vi "Autonomous Independent.vi"   [LabVIEW 2015]
doc: "This VI is called when autonomous begins, and will automatically be terminated when autonomous ends. You can carry out timed or sensor driven robot movement independently without needing to return to the caller."
uses:
  <vilib>/Rock Robotics/WPI/Relay/WPI_RelayValue.ctl
  <vilib>/Rock Robotics/WPI/Utilities/WPI_GetSetVariantRefNum.vi
  <vilib>/Rock Robotics/Network Tables/NT Read String.vi
  <vilib>/Rock Robotics/Network Tables/NT Read Number.vi
  <vilib>/Rock Robotics/Network Tables/NT Write Numeric Array.vi
panel:
  # "Be sure to right-click and choose Data Operations>>Make Current Value default if you want to save the array values with the VI"
types:
  T1 = typedef "WPI_JoystickDevRef.ctl" = cluster{"Device":T2}
  T2 = typedef "WPI_JoystickDeviceEnum.ctl" = enum16{"USB 0", "USB 1", "USB 2", "USB 3", "USB 4", "USB 5"}
  T3 = typedef "WPI_ServoDeviceRef.ctl" = cluster{"DeviceStatus":errorcluster, "PWM Channel":T4, "DeadBand":T5}
  T4 = typedef "FPGA_DIOPWMChannel.ctl" = enum8{"PWM 0", "PWM 1", "PWM 2", "PWM 3", "PWM 4", "PWM 5", "PWM 6", "PWM 7", "PWM 8", "PWM 9", "PWM MXP 0", "PWM MXP 1", "PWM MXP 2", "PWM MXP 3", "PWM MXP 4", "PWM MXP 5", "PWM MXP 6", "PWM MXP 7", "PWM MXP 8", "PWM MXP 9", "Invalid"}
  T5 = typedef "WPI_PWMDeadband.ctl" = cluster{"Name":string, "maxPositivePwm":i32, "minPositivePwm":i32, "centerPwm":i32, "maxNegativePwm":i32, "minNegativePwm":i32, "angularRange":u16}
  T6 = typedef "WPI_RelayValue.ctl" = enum16{"Off", "On", "Forward", "Reverse"}
  T7 = typedef "WPI_SwitchDevRef.ctl" = cluster{"DevStatus":errorcluster, "DIO Channel":T8, "CntIndex":T9, "Normally Closed":bool}
  T8 = typedef "FPGA_DIOChannel.ctl" = enum8{"DIO 0", "DIO 1", "DIO 2", "DIO 3", "DIO 4", "DIO 5", "DIO 6", "DIO 7", "DIO 8", "DIO 9", "DIO MXP 0", "DIO MXP 1", "DIO MXP 2", "DIO MXP 3", "DIO MXP 4", "DIO MXP 5", "DIO MXP 6", "DIO MXP 7", "DIO MXP 8", "DIO MXP 9", "DIO MXP 10", "DIO MXP 11", "DIO MXP 12", "DIO MXP 13", "DIO MXP 14", "DIO MXP 15", "Invalid"}
  T9 = typedef "FPGA_CounterCtrSystemIndex.ctl" = enum8{"Ctr 0", "Ctr 1", "Ctr 2", "Ctr 3", "Ctr 4", "Ctr 5", "Ctr 6", "Ctr 7", "Invalid"}
  T10 = typedef "WPI_RelayDevRef.ctl" = cluster{"DevStatus":errorcluster, "Relay Channel":T11, "Relay Direction":T12}
  T11 = typedef "FPGA_DIORelayChannel.ctl" = enum8{"Relay 0", "Relay 1", "Relay 2", "Relay 3", "Invalid"}
  T12 = typedef "WPI_RelayDirection.ctl" = enum16{"Both directions", "Forward only", "Reverse only"}
  T13 = typedef "WPI_RobotDriveDevRef.ctl" = cluster{"DevStatus":errorcluster, "Motors[]":T14[], "Square Inputs":bool, "Max Output":dbl}
  T14 = typedef "WPI_MotorControlDeviceRef.ctl" = cluster{"DeviceStatus":errorcluster, "Type":T15, "PWM":cluster{"PWM Channel":T4, "DeadBand":T5}, "CAN":cluster{"Device Number":u8, "Control Mode":T16, "Semaphore":T17, "Max Vout":dbl, "TalonSRX Control Mode":T18}, "Invert":bool}
  T15 = typedef "WPI_MotorControlType.ctl" = enum16{"PWM", "CAN", "CANTalonSRX"}
  T16 = typedef "WPI_CANJaguar_ControlMode.ctl" = enum8{"Percent VBus", "Current", "Speed", "Position", "Voltage"}
  T17 = typedef "Semaphore RefNum" = refnum<k1>
  T18 = typedef "WPI_CANTalonSRX_APIControlMode.ctl" = enum8{"Percent VBus", "Speed", "Position", "Slave", "Unchanged / Invalid", "Voltage Compensation", "Current", "Motion Profile"}
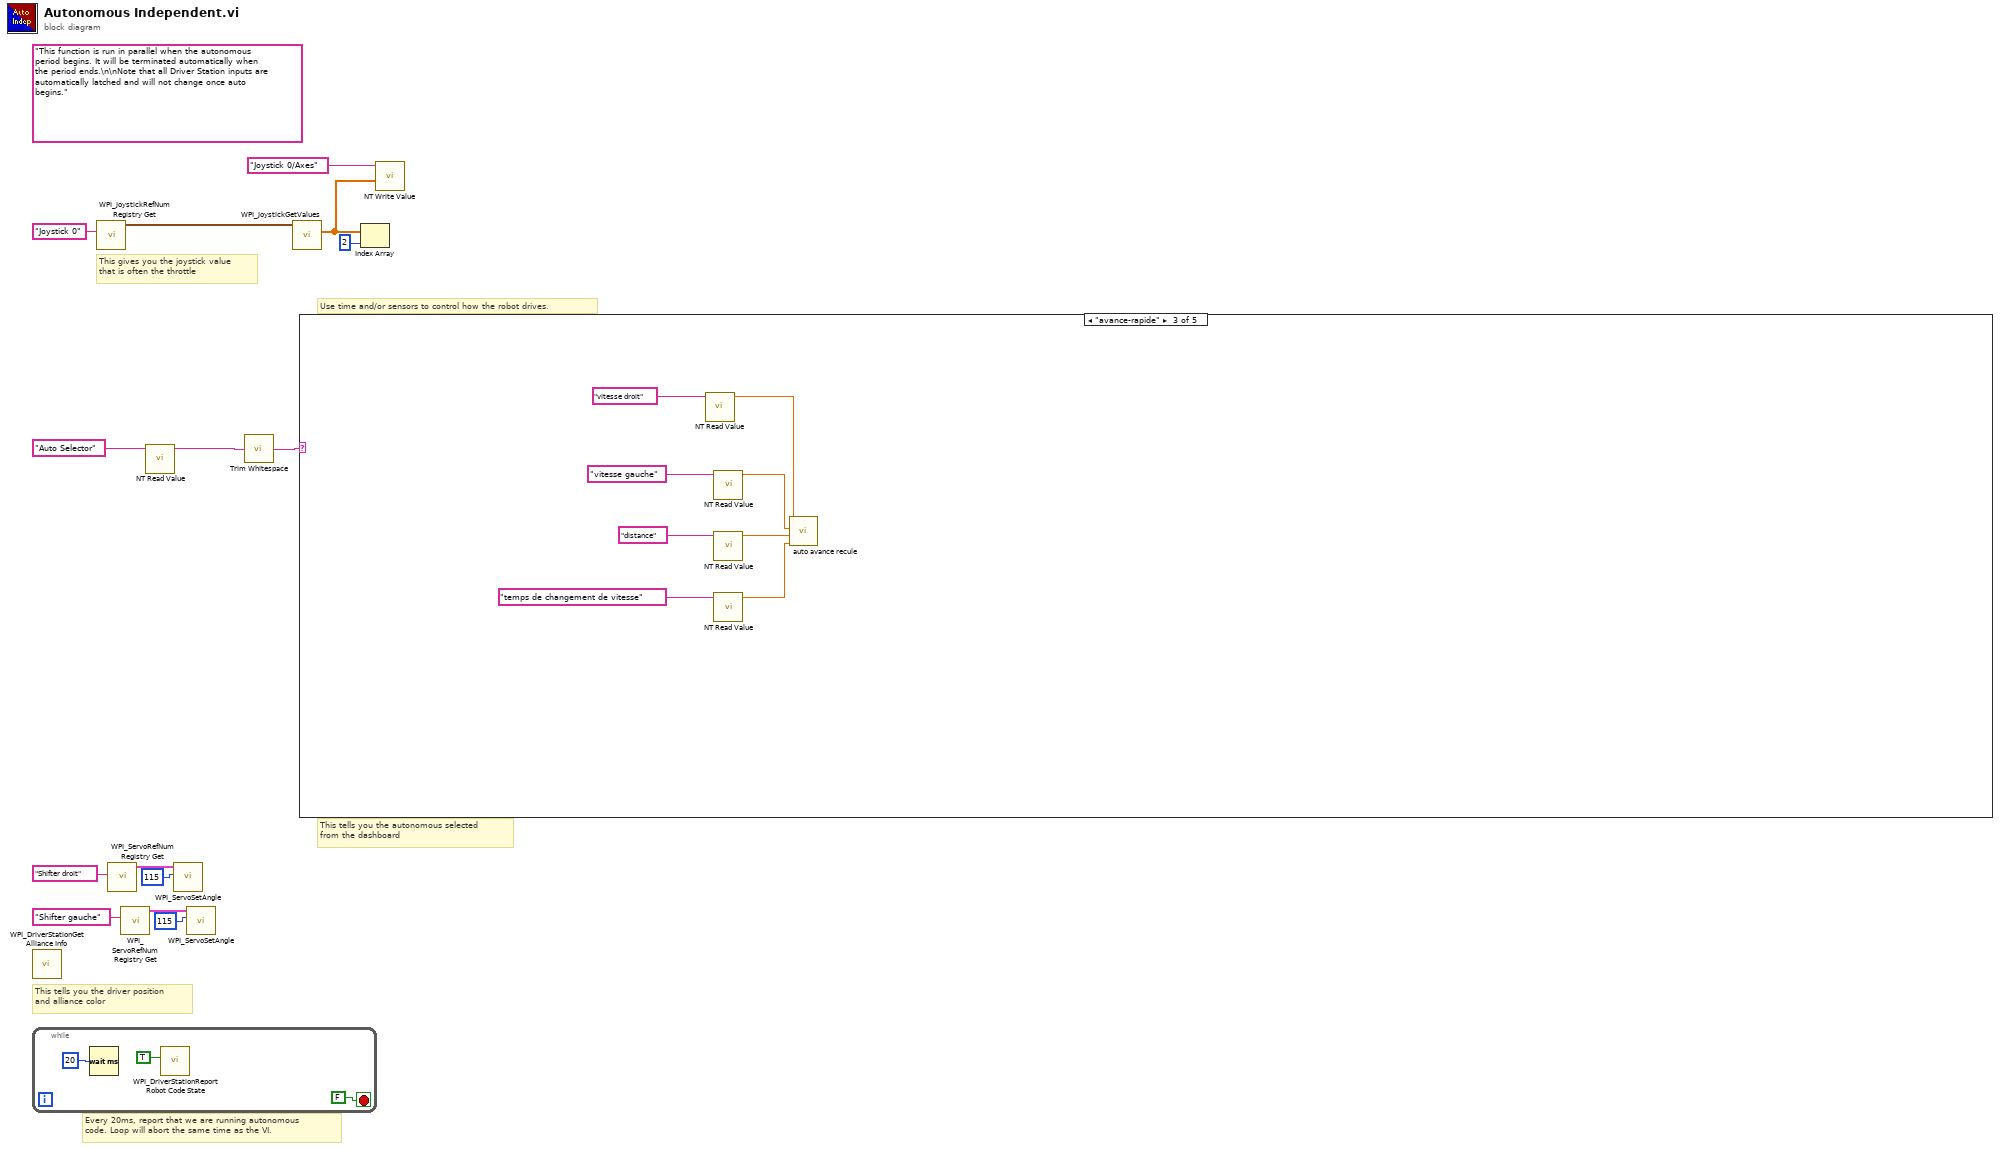
[diagram p0: block diagram]
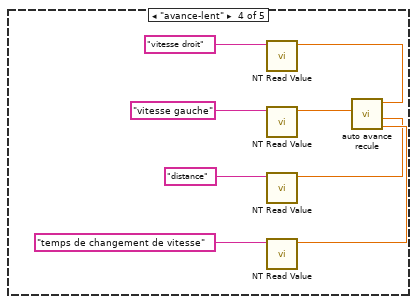
[diagram p4: hidden frame]
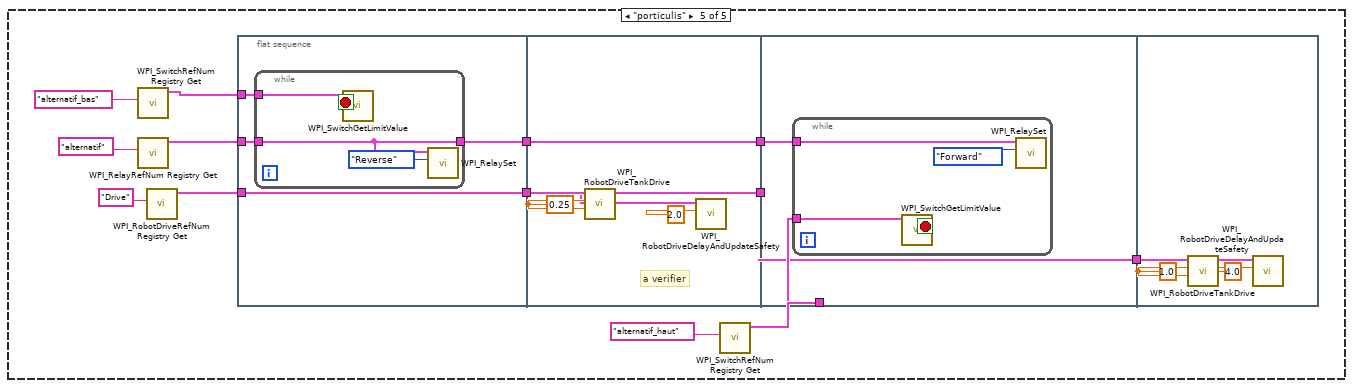
[diagram p5: hidden frame]
diagram:
  (unwired) "This function is run in parallel when the autonomous period begins. It will be terminated automatically when the period ends.\n\nNote that all Driver Station inputs are automatically latched and will not change once auto begins."
  # "This tells you the autonomous selected\nfrom the dashboard"
  # "Every 20ms, report that we are running autonomous\ncode. Loop will abort the same time as the VI."
  # "This gives you the joystick value\nthat is often the throttle"
  # "Use time and/or sensors to control how the robot drives."
  # "This tells you the driver position\nand alliance color"
  n1 = call <vilib>:"WPI_DriverStationGet Alliance Info.vi"() -> ()  [unwired: 12 out]
  n2 = while {
    stop <- FALSE stop-if-true
    n3 = Wait (ms)(milliseconds to wait=u32 20) -> ()  [unwired: 1 out]
    n4 = call <vilib>:"WPI_DriverStationReport Robot Code State.vi"("Autonomous"=TRUE) -> ()  [unwired: 10 in, 1 out]
  }
  n5 = call <vilib>:"WPI_JoystickRefNum Registry Get.vi"("refnum name"="Joystick 0") -> ("JoystickDevRef"=w13:T1)  [unwired: 1 in, 9 out]
  n6 = call <vilib>:"WPI_ServoRefNum Registry Get.vi"("refnum name"="Shifter droit") -> ("ServoDeviceRef"=w5:T3)  [unwired: 9 in, 1 out]
  n7 = call <vilib>:"WPI_ServoRefNum Registry Get.vi"("refnum name"="Shifter gauche") -> ("ServoDeviceRef"=w3:T3)  [unwired: 9 in, 1 out]
  n8 = call-poly <vilib>:"NT Read Value.vi"("Name"="Auto Selector") -> ("String"=w1:string)  [unwired: 9 in, 1 out]
  n9 = call <vilib>:"WPI_ServoSetAngle.vi"("Angle"=115, "ServoDeviceRef"=w5) -> ()  [unwired: 8 in, 2 out]
  n10 = call <vilib>:"WPI_ServoSetAngle.vi"("Angle"=115, "ServoDeviceRef"=w3) -> ()  [unwired: 8 in, 2 out]
  n11 = call <vilib>:"Trim Whitespace.vi"("string"=w1) -> ("trimmed string"=w2:string)  [unwired: 1 in]
  n12 = call <vilib>:"WPI_JoystickGetValues.vi"("JoystickDevRef"=w13) -> ("Axes"=w10:dbl[])  [unwired: 6 in, 4 out]
  n13 = case shown="\"avance-rapide\"" w2 {
    frame Default {
      # "You can put your main auto here, or you can right-click on the case and make any\nother frame be the default case."
      # "This is the frame that will execute if no selection is made, or if it is not recognized"
    }
    frame "rien" {
    }
    frame "avance-rapide" {
      n14 = call-poly <vilib>:"NT Read Value.vi"("Name"="vitesse droit") -> ("Numeric"=w18:dbl)  [unwired: 9 in, 1 out]
      n15 = call-poly <vilib>:"NT Read Value.vi"("Name"="vitesse gauche") -> ("Numeric"=w25:dbl)  [unwired: 9 in, 1 out]
      n16 = call-poly <vilib>:"NT Read Value.vi"("Name"="distance") -> ("Numeric"=w20:dbl)  [unwired: 9 in, 1 out]
      n17 = call-poly <vilib>:"NT Read Value.vi"("Name"="temps de changement de vitesse") -> ("Numeric"=w21:dbl)  [unwired: 9 in, 1 out]
      n18 = call "auto avance recule.vi"("temps de changement de direction"=w21, "temps"=w20, "vitesse gauche"=w25, "vitesse droit"=w18) -> ()  [unwired: 8 in]
    }
    frame "avance-lent" {
      n19 = call-poly <vilib>:"NT Read Value.vi"("Name"="vitesse droit") -> ("Numeric"=w27:dbl)  [unwired: 9 in, 1 out]
      n20 = call-poly <vilib>:"NT Read Value.vi"("Name"="vitesse gauche") -> ("Numeric"=w26:dbl)  [unwired: 9 in, 1 out]
      n21 = call-poly <vilib>:"NT Read Value.vi"("Name"="distance") -> ("Numeric"=w30:dbl)  [unwired: 9 in, 1 out]
      n22 = call-poly <vilib>:"NT Read Value.vi"("Name"="temps de changement de vitesse") -> ("Numeric"=w31:dbl)  [unwired: 9 in, 1 out]
      n23 = call "auto avance recule.vi"("temps de changement de direction"=w31, "temps"=w30, "vitesse gauche"=w26, "vitesse droit"=w27) -> ()  [unwired: 8 in]
    }
    frame "porticulis" {
      n24 = call <vilib>:"WPI_SwitchRefNum Registry Get.vi"("refnum name"="alternatif_bas") -> ("SwitchDevRef"=w40:T7)  [unwired: 9 in, 1 out]
      n25 = call <vilib>:"WPI_RelayRefNum Registry Get.vi"("refnum name"="alternatif") -> ("RelayDevRef"=w42:T10)  [unwired: 9 in, 1 out]
      n26 = call <vilib>:"WPI_RobotDriveRefNum Registry Get.vi"("refnum name"="Drive") -> ("RobotDriveDevRef"=w45:T13)  [unwired: 9 in, 1 out]
      n27 = flat-sequence {
        tunnel: w45 -> [w50]
        tunnel: [w50] -> w44
        tunnel: w42 -> [w49]
        tunnel: w40 -> [w48]
        tunnel: [w47] -> w37
        tunnel: w44 -> [w59]
        tunnel: w37 -> [w56]
        tunnel: [w56] -> w36
        tunnel: [w55] -> w35
        tunnel: w38 -> [w62]
        tunnel: w36 -> [w61]
        tunnel: w35 -> [w60]
        tunnel: [w60] -> w34
        tunnel: w34 -> [w67]
        frame #0 {
          n28 = while {
            tunnel: w49 -> [w51]
            tunnel: w48 -> [w53]
            tunnel: [w51] -> w47
            stop <- w52 stop-if-true
            n29 = call <vilib>:"WPI_SwitchGetLimitValue.vi"("SwitchDevRef"=w53) -> ("Switch Pressed"=w52:bool)  [unwired: 8 in, 2 out]
            n30 = call <vilib>:"WPI_RelaySet.vi"("RelayValue"=WPI_RelayValue."Reverse", "RelayDevRef"=w51) -> ()  [unwired: 8 in, 2 out]
          }
        }
        frame #1 {
          w58 = 0.25 ("Left axis value")
          # "a verifier"
          n31 = call <vilib>:"WPI_RobotDriveTankDrive.vi"("Right axis value"=w58, "Left axis value"=w58, "RobotDriveDevRef"=w59) -> ("RobotDriveDevRef"=w55:T13)  [unwired: 6 in, 2 out]
          n32 = call <vilib>:"WPI_RobotDriveDelayAndUpdateSafety.vi"("Delay (s)"=2.0, "RobotDriveDevRef"=w55) -> ()  [unwired: 8 in, 2 out]
        }
        frame #2 {
          n33 = while {
            tunnel: w61 -> [w65]
            tunnel: w62 -> [w64]
            stop <- w63 stop-if-true
            n34 = call <vilib>:"WPI_SwitchGetLimitValue.vi"("SwitchDevRef"=w64) -> ("Switch Pressed"=w63:bool)  [unwired: 8 in, 2 out]
            n35 = call <vilib>:"WPI_RelaySet.vi"("RelayValue"=WPI_RelayValue."Forward", "RelayDevRef"=w65) -> ()  [unwired: 8 in, 2 out]
          }
        }
        frame #3 {
          w69 = 1.0 ("Left axis value")
          n36 = call <vilib>:"WPI_RobotDriveTankDrive.vi"("Right axis value"=w69, "Left axis value"=w69, "RobotDriveDevRef"=w67) -> ("RobotDriveDevRef"=w70:T13)  [unwired: 6 in, 2 out]
          n37 = call <vilib>:"WPI_RobotDriveDelayAndUpdateSafety.vi"("Delay (s)"=4.0, "RobotDriveDevRef"=w70) -> ()  [unwired: 8 in, 2 out]
        }
      }
      n38 = call <vilib>:"WPI_SwitchRefNum Registry Get.vi"("refnum name"="alternatif_haut") -> ("SwitchDevRef"=w38:T7)  [unwired: 9 in, 1 out]
    }
  }
  n39 = Index Array(array=w10, index=2) -> ()  [unwired: 1 out]
  n40 = call-poly <vilib>:"NT Write Value.vi"("Numeric Array"=w10, "Name"="Joystick 0/Axes") -> ()  [unwired: 9 in, 1 out]
